vi "Send-valve-interface.vi"(8 "error in (no error)":errorcluster, 10 "Valves":bool[](array[boolean])) -> (0 "error out":errorcluster)   [LabVIEW 2021, in "Valve-Module.lvlib"]
doc: "_______\nCreated using Delacor User Event Scripter 1.0.0.6."
uses:
  Valve-Module.lvlib
  Send-valve-interface Argument--cluster.ctl
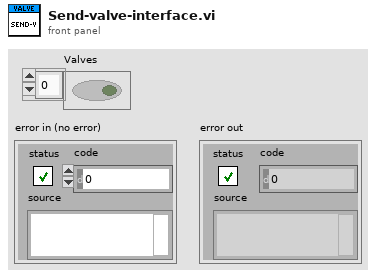
[diagram p1: front panel]
types:
  T1 = typedef "Valve-Module.lvlib/Send-valve-interface Argument--cluster.ctl" = cluster{"Valves":bool[]}
  T2 = typedef "Valve-Module.lvlib/Broadcast Events--cluster.ctl" = cluster{"Status Updated":refnum<user-event>, "Send-valve-interface":refnum<user-event>}
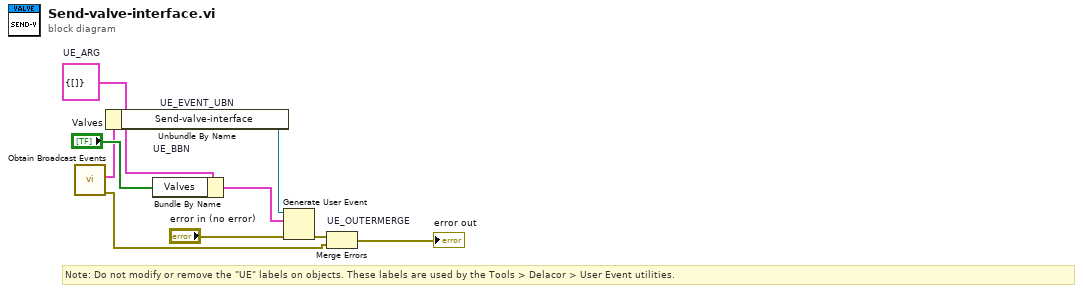
[diagram p0: block diagram]
diagram:
  w4 = T1 {"Valves"=[]}  # UE_ARG
  # "Note: Do not modify or remove the \"UE\" labels on objects. These labels are used by the Tools > Delacor > User Event utilities."
  n1 = call "Obtain Broadcast Events.vi"() -> ("error out"=w2:errorcluster, "Valve-Module Broadcast Events"=w1:T2)  [unwired: 10 in]
  n2 = Unbundle By Name "UE_EVENT_UBN"(w1) -> ("Send-valve-interface"=w6:refnum<user-event>)
  n3 = Bundle By Name "UE_BBN"(cluster=w4, "Valves"="Valves") -> (w7:T1)
  n4 = Generate User Event(user event=w6, event data cluster=w7, error in="error in (no error)") -> (error out=w5:errorcluster)  [unwired: 1 in, 1 out]
  n5 = Merge Errors "UE_OUTERMERGE"(w5, w2) -> (→"error out":errorcluster)
